vi "translate raw memory to NI Image.vi"(7 "Image in":T2, 8 "error in (no error)":errorcluster, 9 "pBuffer":u8[](array[numeric]), 10 "LIMPICTURE in":T1, 11 "hFile in":T3) -> (0 "error out":errorcluster, 2 "LIMPICTURE out":T1, 3 "hFile out":T3, 5 "Image out":T2)   [LabVIEW 2014, in "ND2_Reader_32.lvlib"]
uses:
  ND2_Reader_32.lvlib
  controls/numeric_LIMFILEHANDLE.ctl
  controls/cluster_LIMPICTURE.ctl
  <vilib>/vision/Image Controls.llb/IMAQ Image.ctl
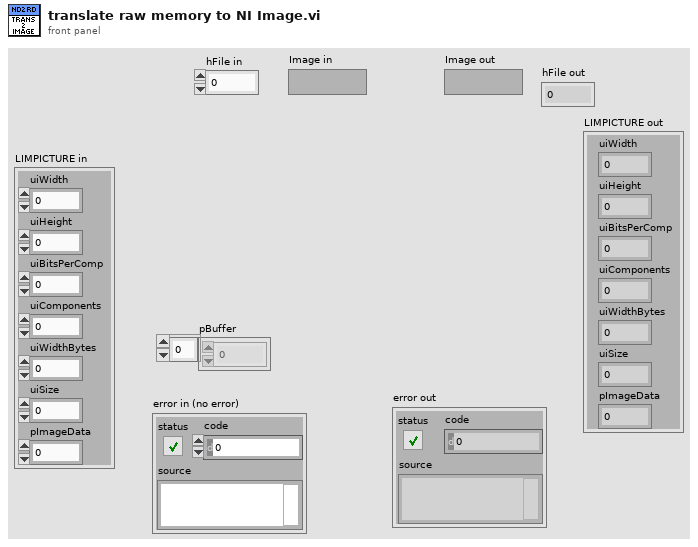
[diagram p1: front panel]
types:
  T1 = typedef "cluster_LIMPICTURE.ctl" = cluster{"uiWidth":u32, "uiHeight":u32, "uiBitsPerComp":u32, "uiComponents":u32, "uiWidthBytes":u32, "uiSize":u32, "pImageData":u32}
  T2 = typedef "IMAQ Image.ctl" = refnum<image>
  T3 = typedef "numeric_LIMFILEHANDLE.ctl" = i32
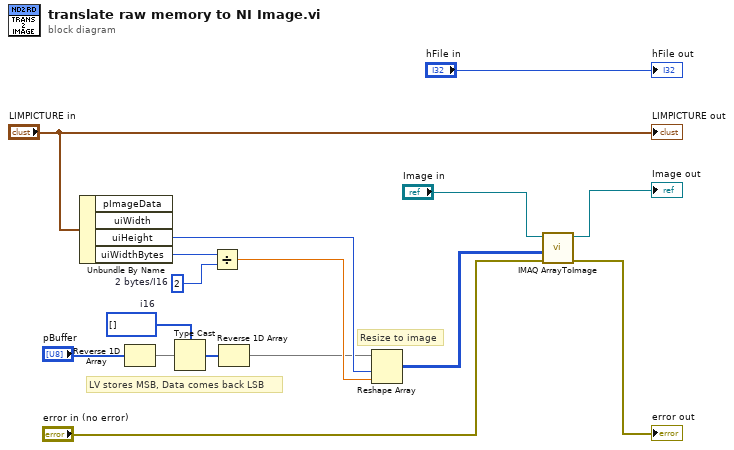
[diagram p0: block diagram]
diagram:
  w12 = u32 2  # 2 bytes/I16
  w14 = i16[] []  # i16
  # "Resize to image"
  # "LV stores MSB, Data comes back LSB"
  n1 = Unbundle By Name("LIMPICTURE in") -> ("uiHeight"=w10:u32, "uiWidthBytes"=w13:u32)  [unwired: 2 out]
  n2 = Reverse 1D Array(array="pBuffer") -> (reversed array=w8:u8[])
  n3 = Type Cast(type=w14, x=w8) -> (*(type *) &x=w11:i16[])
  n4 = Divide(x=w13, y=w12) -> (x/y=w9:dbl)
  n5 = Reverse 1D Array(array=w11) -> (reversed array=w7:i16[])
  n6 = Reshape Array(w7, w10, w9) -> (w5:i16[][])
  n7 = call "IMAQ ArrayToImage"("error in (no error)"="error in (no error)", "Image Pixels (I16)"=w5, "Image"="Image in") -> ("error out"=→"error out":errorcluster, "Image Out"=→"Image out":T2)  [unwired: 7 in]
  "hFile out" <- "hFile in"
  "LIMPICTURE out" <- "LIMPICTURE in"
